vi "Search_dust_names.vi"(8 "error in (no error)":errorcluster, 11 "Dust array in":T1[](array[typedef])) -> (0 "error out":errorcluster, 2 "Cancelled?":bool, 3 "Dust array out":T1[](array[typedef]))   [LabVIEW 2013]
doc: "Sub-vi of Search_Dust_Type. Selects rows from the dust_type table by dust name."
uses:
  <userlib>/Accelerator/User Interface/Controls/Dust_list.ctl
  <vilib>/Utility/miscctls.llb/LVPointTypeDef.ctl
panel:
  in  "Get All":bool
  in  "Cancel":bool
  in  "Select":bool
  in  "Search":bool
  in  "Search Name":string
  out "Dust Name Array":string[](array[string])
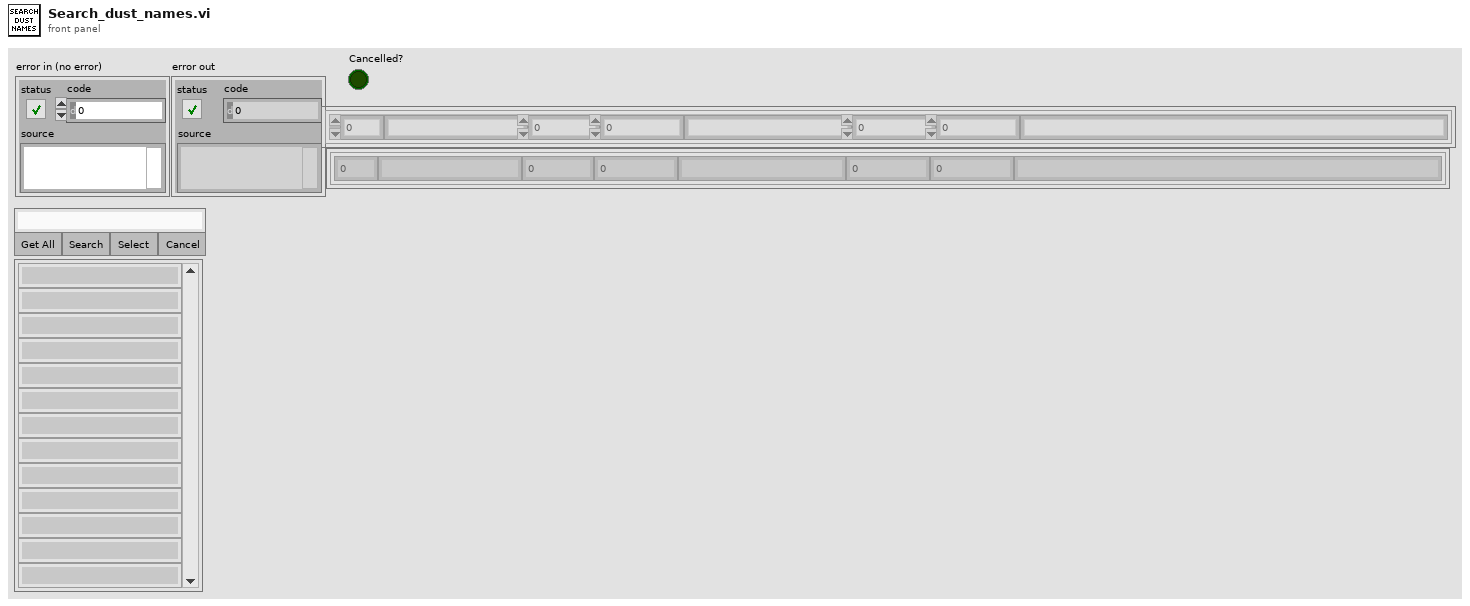
[diagram p1: front panel]
types:
  T1 = typedef "Dust_list.ctl" = cluster{"id_dust_type":i32, "dust_name":string, "dust_type":i32, "batch_no":i32, "dust_density":dbl, "source_weight":dbl, "size":string, "bottle_weight":dbl, "dust_mass":dbl, "comments":string}
  T2 = enum16{"dust_name", "dust_density", "source_weight", "bottle_weight", "dust_weight"}
  T3 = typedef "LVPointTypeDef.ctl" = cluster{"Horizontal":i16, "Vertical":i16}
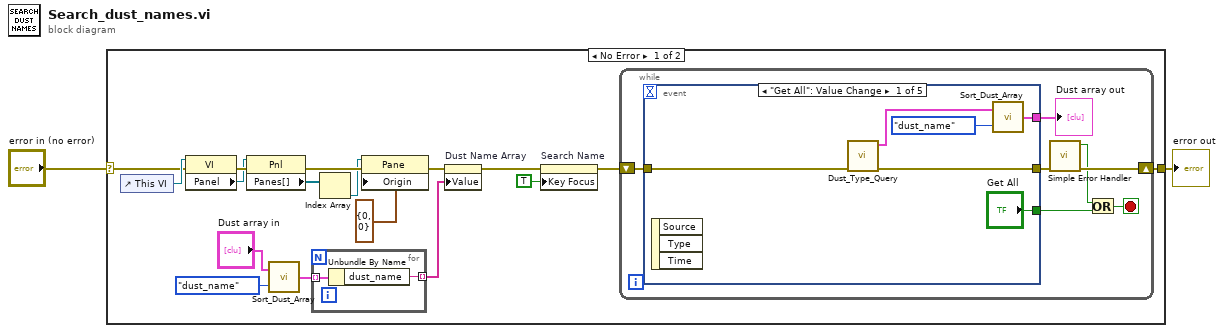
[diagram p0: block diagram]
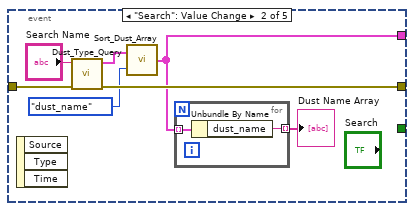
[diagram p2: hidden frame]
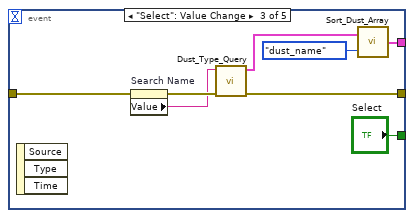
[diagram p3: hidden frame]
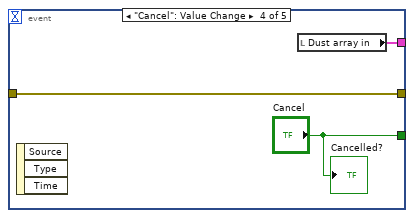
[diagram p4: hidden frame]
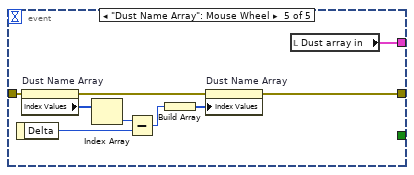
[diagram p5: hidden frame]
diagram:
  n1 = case shown="No Error" "error in (no error)" {
    selector: "error in (no error)" -> [w11 w64]
    tunnel: [w10 w64] -> w1
    frame No Error {
      n2 = control-ref of="This VI"() -> (w18:refnum<vi>)
      n3 = property class="VI"(reference=w18, error in=w11) -> (error out=w17:errorcluster, "Panel"=w16:refnum<vi>)  [unwired: 1 out]
      n4 = property class="Pnl"(reference=w16, error in=w17) -> (error out=w15:errorcluster, "Panes[]"=w14:refnum<vi>[])  [unwired: 1 out]
      n5 = call <userlib>:"Sort_Dust_Array.vi"("Order by..."=T2."dust_name", "Array In"="Dust array in") -> ("Array out"=w7:T1[])
      n6 = for {
        tunnel: w7 -> [w63] mode=indexing
        tunnel: [w62] -> w9 mode=indexing
        n7 = Unbundle By Name(w63) -> ("dust_name"=w62:string)
      }
      n8 = Index Array(array=w14) -> (element=w13:refnum<vi>)  [unwired: 1 in]
      n9 = property class="Pane"(reference=w13, error in=w15, "Origin"=T3 {"Horizontal"=0, "Vertical"=0}) -> (error out=w19:errorcluster)  [unwired: 1 out]
      n10 = property on="Dust Name Array" class="Arr (strict)"(error in=w19, "Value"=w9) -> (error out=w4:errorcluster)  [unwired: 1 in, 1 out]
      n11 = property on="Search Name" class="Str"(error in=w4, "Key Focus"=TRUE) -> (error out=w3:errorcluster)  [unwired: 1 in, 1 out]
      n12 = while {
        shift-right: [w24] -> w10
        shift-left: w3 -> [w20]
        stop <- w23 stop-if-true
        n13 = event shown="[0] \"Get All\": Value Change" {
          selector: _ -> [_ _ _ _ _]
          dyn-events: _ -> [_ _ _ _ _]
          timeout: _ -> [_ _ _ _ _]
          tunnel: [w31 w39 w48 w52 w57] -> w26
          tunnel: w20 -> [w32 w37 w45 w52 w61]
          tunnel: ["Get All" _ "Select" "Cancel" _] -> w25
          tunnel: [w28 w33 w43 w50 w54] -> w21
          event "Get All": Value Change {
            n14 = event-data() -> ()  [unwired: 1 in, 3 out]
            n15 = call <userlib>:"Dust_Type_Query.vi"("error in (no error)"=w32) -> ("error out"=w31:errorcluster, "Dust Type Array"=w27:T1[])  [unwired: 9 in]
            n16 = call <userlib>:"Sort_Dust_Array.vi"("Order by..."=T2."dust_name", "Array In"=w27) -> ("Array out"=w28:T1[])
          }
          event "Search": Value Change {
            n17 = event-data() -> ()  [unwired: 1 in, 3 out]
            n18 = call <userlib>:"Dust_Type_Query.vi"("error in (no error)"=w37, "Dust Name"="Search Name") -> ("error out"=w39:errorcluster, "Dust Type Array"=w34:T1[])  [unwired: 8 in]
            n19 = call <userlib>:"Sort_Dust_Array.vi"("Order by..."=T2."dust_name", "Array In"=w34) -> ("Array out"=w33:T1[])
            n20 = for {
              tunnel: [w41] -> w36 mode=indexing
              tunnel: w33 -> [w40] mode=indexing
              n21 = Unbundle By Name(w40) -> ("dust_name"=w41:string)
            }
            "Dust Name Array" <- w36
          }
          event "Select": Value Change {
            n22 = event-data() -> ()  [unwired: 1 in, 3 out]
            n23 = property on="Search Name" class="Str"(error in=w45) -> (error out=w47:errorcluster, "Value"=w46:string)  [unwired: 1 in, 1 out]
            n24 = call <userlib>:"Dust_Type_Query.vi"("error in (no error)"=w47, "Dust Name"=w46) -> ("error out"=w48:errorcluster, "Dust Type Array"=w42:T1[])  [unwired: 8 in]
            n25 = call <userlib>:"Sort_Dust_Array.vi"("Order by..."=T2."dust_name", "Array In"=w42) -> ("Array out"=w43:T1[])
          }
          event "Cancel": Value Change {
            n26 = event-data() -> ()  [unwired: 1 in, 3 out]
            n27 = local read "Dust array in"() -> (w50:T1[])
            "Cancelled?" <- "Cancel"
          }
          event "Dust Name Array": Mouse Wheel {
            n28 = event-data() -> ("Delta"=w60:i32)  [unwired: 1 in]
            n29 = property on="Dust Name Array" class="Arr (strict)"(error in=w61) -> (error out=w58:errorcluster, "Index Values"=w56:u32[])  [unwired: 1 in, 1 out]
            n30 = Index Array(array=w56) -> (element=w55:u32)  [unwired: 1 in]
            n31 = Subtract(x=w55, y=w60) -> (x-y=w53:u32)
            n32 = Build Array(w53) -> (w59:u32[])
            n33 = property on="Dust Name Array" class="Arr (strict)"(error in=w58, "Index Values"=w59) -> (error out=w57:errorcluster)  [unwired: 1 in, 1 out]
            n34 = local read "Dust array in"() -> (w54:T1[])
          }
        }
        "Dust array out" <- w21
        n35 = call <vilib>:"Simple Error Handler.vi"("error in (no error)"=w26) -> ("error?"=w22:bool, "error out"=w24:errorcluster)  [unwired: 4 in, 3 out]
        n36 = Or(x=w22, y=w25) -> (x .or. y?=w23:bool)
      }
    }
    frame Error {
    }
  }
  "error out" <- w1
